vi "menu_song_select.vi"(0 "song id":enum16{"0", "1"}(ring), 1 "difficulty":enum16{"easy", "hard"}(ring), 2 "showcase":bool=TRUE, 3 "state change":bool=TRUE, 4 "game state":T1(ring), 5 "timer":dbl, 6 "prepare menu":enum16{"difficulty", "bot"}(ring)) -> (14 "new picture":picture, 17 "animating?":bool)   [LabVIEW 2023]
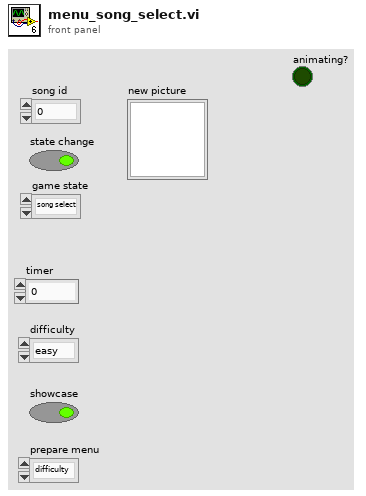
[diagram p1: front panel]
types:
  T1 = enum16{"song select", "difficulty select", "gameplay", "result"}
  T2 = cluster{"Width":i16, "Style":enum32{"Solid", "Dash", "Dot", "DashDot", "DashDotDot"}}
  T3 = cluster{"Width":u16, "Style":enum32{"Solid", "Dash", "Dot", "DashDot", "DashDotDot"}}
  T4 = cluster{"horizontal":enum16{"left", "center", "right"}, "vertical":enum16{"top", "center", "bottom"}}
  T5 = cluster{"Font Name:":string, "Size":i16, "Strikeout?":bool, "Italic?":bool, "Underline?":bool, "Outline?":bool, "Shadow?":bool, "Bold?":bool}
  T6 = enum16{"User-specified Font", "Application Font", "System Font", "Dialog Font"}
  T7 = enum16{"None", "Stacked", "Clockwise", "Counterclockwise"}
  T8 = typedef "imagedata.ctl" = cluster{"image type":i32, "image depth":i32, "image":u8[], "mask":u8[], "colors":u32[], "Rectangle":cluster{"left":i16, "top":i16, "right":i16, "bottom":i16}}
  T9 = cluster{"left":i16, "left":i16, dbl, "bottom":i16}
  T10 = cluster{dbl, "top":i16, "right":i16, "bottom":i16}
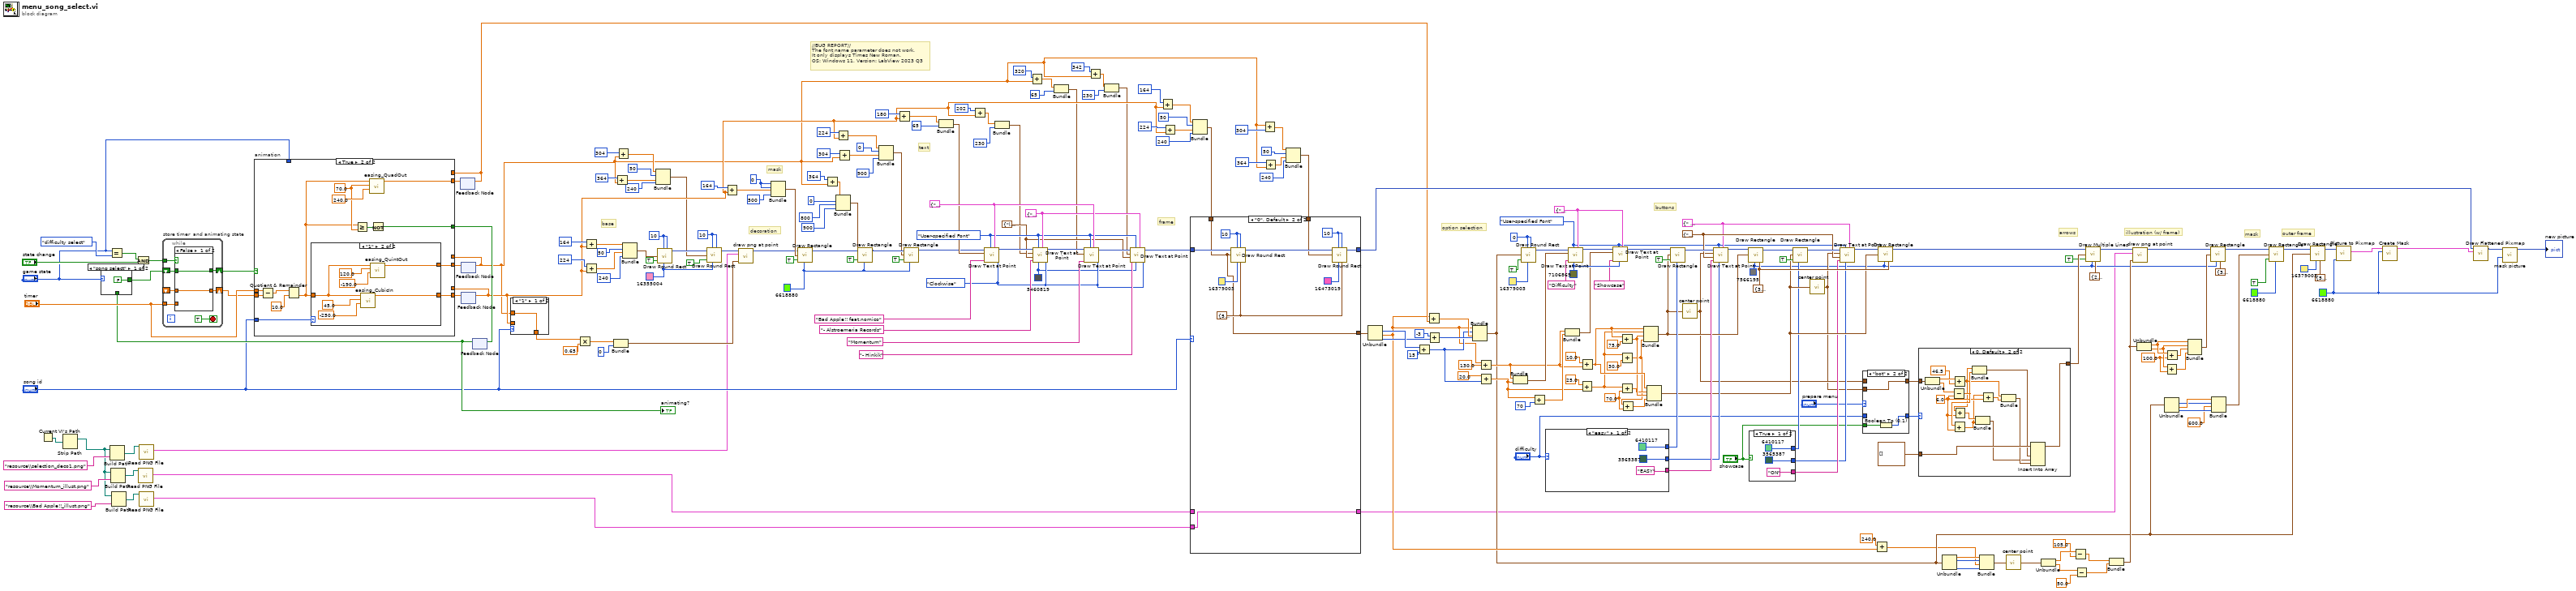
[diagram p0: block diagram]
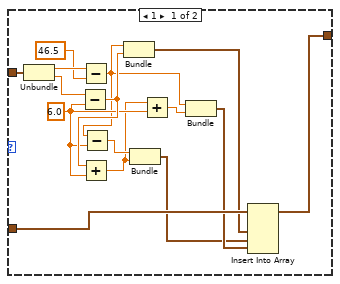
[diagram p2: hidden frame]
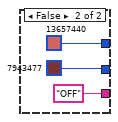
[diagram p4: hidden frame]
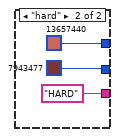
[diagram p5: hidden frame]
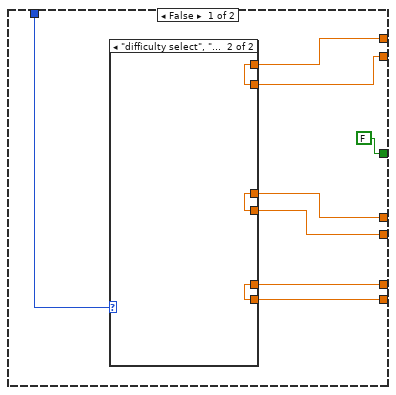
[diagram p7: hidden frame]
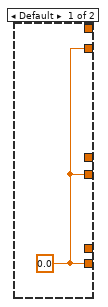
[diagram p8: hidden frame]
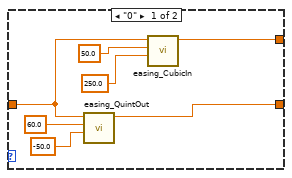
[diagram p9: hidden frame]
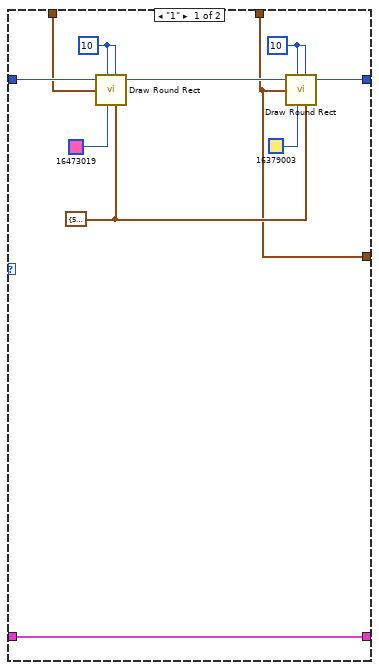
[diagram p12: hidden frame]
diagram:
  w47 = 100.0 ("y")
  w85 = 70.0 ("x")
  w80 = T4 {"horizontal"=enum."center", "vertical"=enum."center"} ("alignment(left, top)")
  w78 = T5 {"Font Name:"=" ", "Size"=15, "Strikeout?"=FALSE, "Italic?"=FALSE, "Underline?"=FALSE, "Outline?"=FALSE, "Shadow?"=FALSE, "Bold?"=TRUE} ("[user-specified font]")
  w81 = T2 {"Width"=3, "Style"=enum."DashDotDot"} ("pen")
  w43 = u32 7566195 ("color(black)")
  w106 = u32 5460819 ("text color(black)")
  w112 = u32 7106869 ("text color(black)")
  w77 = T6."User-specified Font" ("desired font(Application)")
  w113 = T5 {"Font Name:"="a", "Size"=16, "Strikeout?"=FALSE, "Italic?"=FALSE, "Underline?"=FALSE, "Outline?"=FALSE, "Shadow?"=FALSE, "Bold?"=TRUE} ("[user-specified font]")
  w120 = i16 0
  w176 = T7."Clockwise" ("text orientation")
  w197 = i16 0 ("left")
  w221 = T5 {"Font Name:"="k", "Size"=13, "Strikeout?"=FALSE, "Italic?"=TRUE, "Underline?"=FALSE, "Outline?"=FALSE, "Shadow?"=FALSE, "Bold?"=TRUE} ("[user-specified font]")
  w219 = T4 {"horizontal"=enum."left", "vertical"=enum."bottom"} ("alignment(left, top)")
  w222 = T5 {"Font Name:"="Arial", "Size"=15, "Strikeout?"=FALSE, "Italic?"=FALSE, "Underline?"=FALSE, "Outline?"=FALSE, "Shadow?"=FALSE, "Bold?"=TRUE} ("[user-specified font]")
  w220 = T6."User-specified Font" ("desired font(Application)")
  w29 = u32 6618880 ("color(black)")
  w18 = u32 6618880 ("color(black)")
  w235 = i16 10
  w236 = i16 10
  w234 = u32 16355004 ("color(black)")
  # "outer frame"
  # "mask"
  # "illustration (w/ frame)"
  # "arrows"
  # "buttons"
  # "//BUG REPORT//\nThe font name parameter does not work.\nIt only displays Times New Roman.\nOS: Windows 11, Version: LabView 2023 Q3"
  # "option selection"
  # "frame"
  # "text"
  # "mask"
  # "decoration"
  # "base"
  n1 = Current VI's Path() -> (path=w14:path)
  n2 = Strip Path(path=w14) -> (stripped path=w11:path)  [unwired: 1 out]
  n3 = Equal?(x="game state", y=T1."difficulty select" ("game state 2")) -> (x = y?=w215:bool)
  n4 = Build Path(base path=w11, name or relative path="resource\\selection_deco1.png") -> (appended path=w9:path)
  n5 = Build Path(base path=w11, name or relative path="resource\\Momentum_illust.png") -> (appended path=w7:path)
  n6 = Build Path(base path=w11, name or relative path="resource\\Bad Apple!!_illust.png") -> (appended path=w5:path)
  n7 = And(x=w215, y="state change") -> (x .and. y?=w214:bool)
  n8 = call <vilib>:"Read PNG File.vi"("path to PNG file"=w7) -> ("image data"=w6:T8)  [unwired: 8 in, 2 out]
  n9 = call <vilib>:"Read PNG File.vi"("path to PNG file"=w5) -> ("image data"=w4:T8)  [unwired: 8 in, 2 out]
  n10 = call <vilib>:"Read PNG File.vi"("path to PNG file"=w9) -> ("image data"=w8:T8)  [unwired: 8 in, 2 out]
  n11 = feedback #1() -> (w37:dbl)  [unwired: 1 in]
  n12 = feedback #2() -> (w130:dbl)  [unwired: 1 in]
  n13 = feedback #3() -> (w158:dbl)  [unwired: 1 in]
  n14 = feedback #4() -> (w161:bool)  [unwired: 1 in]
  "animating?" <- w161
  n15 = case shown="\"song select\"" "game state" {
    tunnel: [FALSE w240] -> w209
    tunnel: w161 -> [_ w240]
    frame "song select" {
    }
    frame Default {
    }
  }
  n16 = while "store timer  and animating state" {
    tunnel: w214 -> [w246]
    tunnel: "timer" -> [w245]
    shift-right: [w244] -> w210
    shift-left: _ -> [w243]
    shift-right: [w242] -> w203
    shift-left: w209 -> [w241]
    stop <- TRUE stop-if-true
    n17 = case shown="False" w246 {
      selector: w246 -> [_ w250]
      tunnel: w245 -> [_ w251]
      tunnel: [w249 w251] -> w244
      tunnel: w243 -> [w249 _]
      tunnel: [w248 w250] -> w242
      tunnel: w241 -> [w248 _]
      frame False {
      }
      frame True {
      }
    }
  }
  n18 = case "animation" shown="True" w203 {
    tunnel: "timer" -> [_ w276]
    tunnel: w210 -> [_ w275]
    tunnel: [w257 w272] -> w205
    tunnel: w158 -> [w256 _]
    tunnel: [FALSE ("fill?(F)") w264] -> w204
    tunnel: "game state" -> [w258 _]
    tunnel: "song id" -> [_ w271]
    tunnel: [w255 w270] -> w160
    tunnel: w130 -> [w254 _]
    tunnel: [w253 w266] -> w38
    tunnel: w37 -> [w252 _]
    frame False {
      n19 = case shown="\"difficulty select\", \"gameplay\"" w258 {
        tunnel: [w260 w263] -> w257
        tunnel: w256 -> [_ w263]
        tunnel: [w260 w262] -> w255
        tunnel: w254 -> [_ w262]
        tunnel: [w260 w261] -> w253
        tunnel: w252 -> [_ w261]
        frame Default {
          w260 = 0.0
        }
        frame "difficulty select", "gameplay" {
        }
      }
    }
    frame True {
      w268 = 70.0 ("y")
      n20 = Subtract(x=w276, y=w275) -> (x-y=w274:dbl)
      n21 = Quotient & Remainder(x=w274, y=10.0) -> (floor(x/y)=w267:dbl)  [unwired: 1 out]
      n22 = case shown="\"1\"" w271 {
        tunnel: w267 -> [w279 w284]
        tunnel: [w281 w286] -> w272
        tunnel: [w280 w289] -> w270
        frame "0" {
          n23 = call "easing_QuintOut.vi"("distance"=-50.0 ("y"), "interval (10 ms)"=60.0 ("y"), "time"=w279) -> ("current pos"=w281:dbl)  [unwired: 8 in]
          n24 = call "easing_CubicIn.vi"("distance"=250.0 ("y"), "interval (10 ms)"=50.0 ("y"), "time"=w279) -> ("current position"=w280:dbl)  [unwired: 8 in]
        }
        frame "1" {
          n25 = call "easing_CubicIn.vi"("distance"=-250.0 ("y"), "interval (10 ms)"=45.0 ("y"), "time"=w284) -> ("current position"=w286:dbl)  [unwired: 8 in]
          n26 = call "easing_QuintOut.vi"("distance"=-190.0 ("y"), "interval (10 ms)"=120.0 ("y"), "time"=w284) -> ("current pos"=w289:dbl)  [unwired: 8 in]
        }
      }
      n27 = Greater Or Equal?(x=w267, y=w268) -> (x >= y?=w265:bool)
      n28 = call "easing_QuadOut.vi"("distance"=240.0 ("y"), "interval (10 ms)"=w268, "time"=w267) -> ("current pos"=w266:dbl)  [unwired: 8 in]
      n29 = Not(x=w265) -> (.not. x?=w264:bool)
    }
  }
  n30 = feedback-in #1(w38) -> ()
  n31 = feedback-in #2(w160) -> ()
  n32 = feedback-in #3(w205) -> ()
  n33 = feedback-in #4(w204) -> ()
  n34 = case shown="\"1\"" "song id" {
    tunnel: [w291 w292] -> w159
    tunnel: w158 -> [_ w292]
    tunnel: w130 -> [w291 _]
    frame "1" {
    }
    frame "0" {
    }
  }
  n35 = Multiply(x=w159, y=0.65) -> (x*y=w170:dbl)
  n36 = Add(x=i16 164, y=w158) -> (x+y=w198:dbl)
  n37 = Add(x=i16 224, y=w158) -> (x+y=w200:dbl)
  n38 = Bundle(w170, "y"=i16 0) -> (w173:cluster{dbl, "y":i16})  [unwired: 1 in]
  n39 = Add(x=i16 364 ("right"), y=w130) -> (x+y=w151:dbl)
  n40 = Add(x=i16 304 ("left"), y=w130) -> (x+y=w150:dbl)
  n41 = Bundle(w198, i16 50, w200, i16 240) -> (w206:cluster{dbl, i16, dbl, i16})  [unwired: 1 in]
  n42 = Bundle(w150, "top"=i16 50, w151, "bottom"=i16 240) -> (w156:cluster{dbl, "top":i16, dbl, "bottom":i16})  [unwired: 1 in]
  n43 = call <vilib>:"Draw Round Rect.vi"("oval width"=w236, "rect"=w206, "fill?(F)"=TRUE, "color(black)"=w234, "oval height"=w236) -> ("new picture"=w233:picture)  [unwired: 4 in]
  n44 = call <vilib>:"Draw Round Rect.vi"("picture"=w233, "oval width"=w235, "rect"=w156, "fill?(F)"=TRUE, "color(black)"=w234, "oval height"=w235) -> ("new picture"=w174:picture)  [unwired: 3 in]
  n45 = Add(x=i16 164 ("right"), y=w158) -> (x+y=w193:dbl)
  n46 = call "draw png at point.vi"("top left point(0, 0)"=w173, "image data"=w8, "new picture in"=w174) -> ("new picture out"=w175:picture)  [unwired: 8 in]
  n47 = Bundle("left"=w197, "left"=w197, w193, "bottom"=i16 500) -> (w195:T9)  [unwired: 1 in]
  n48 = call <vilib>:"Draw Rectangle.vi"("picture"=w175, "rect"=w195, "fill?(F)"=TRUE, "color(black)"=w29) -> ("new picture"=w230:picture)  [unwired: 5 in]
  n49 = Add(x=i16 364 ("left"), y=w130) -> (x+y=w131:dbl)
  n50 = Add(x=i16 224 ("left"), y=w158) -> (x+y=w177:dbl)
  n51 = Bundle(w131, "top"=i16 0, "right"=i16 800, "bottom"=i16 900) -> (w192:T10)  [unwired: 1 in]
  n52 = Add(x=i16 304 ("right"), y=w130) -> (x+y=w148:dbl)
  n53 = call <vilib>:"Draw Rectangle.vi"("picture"=w230, "rect"=w192, "fill?(F)"=TRUE, "color(black)"=w29) -> ("new picture"=w228:picture)  [unwired: 5 in]
  n54 = Bundle(w177, "top"=i16 0, w148, "bottom"=i16 900) -> (w181:cluster{dbl, "top":i16, dbl, "bottom":i16})  [unwired: 1 in]
  n55 = Add(x=i16 180, y=w158) -> (x+y=w186:dbl)
  n56 = call <vilib>:"Draw Rectangle.vi"("picture"=w228, "rect"=w181, "fill?(F)"=TRUE, "color(black)"=w29) -> ("new picture"=w2:picture)  [unwired: 5 in]
  n57 = Bundle(w186, "y"=i16 65) -> (w188:cluster{dbl, "y":i16})  [unwired: 1 in]
  n58 = Add(x=i16 202, y=w158) -> (x+y=w165:dbl)
  n59 = call <vilib>:"Draw Text at Point.vi"("text orientation"=w176, "[user-specified font]"=w222, "desired font(Application)"=w220, "text"="Bad Apple!! feat.nomico", "origin"=w188, "picture"=w2) -> ("new picture"=w226:picture)  [unwired: 4 in, 1 out]
  n60 = Bundle(w165, "y"=i16 230) -> (w184:cluster{dbl, "y":i16})  [unwired: 1 in]
  n61 = Add(x=i16 320, y=w130) -> (x+y=w144:dbl)
  n62 = call <vilib>:"Draw Text at Point.vi"("text orientation"=w176, "[user-specified font]"=w221, "text color(black)"=w106, "desired font(Application)"=w220, "text"="- Alstroemeria Records", "alignment(left, top)"=w219, "origin"=w184, "picture"=w226) -> ("new picture"=w224:picture)  [unwired: 2 in, 1 out]
  n63 = Bundle(w144, "y"=i16 65) -> (w147:cluster{dbl, "y":i16})  [unwired: 1 in]
  n64 = call <vilib>:"Draw Text at Point.vi"("text orientation"=w176, "[user-specified font]"=w222, "desired font(Application)"=w220, "text"="Momentum", "origin"=w147, "picture"=w224) -> ("new picture"=w223:picture)  [unwired: 4 in, 1 out]
  n65 = Add(x=i16 342, y=w130) -> (x+y=w140:dbl)
  n66 = Bundle(w140, "y"=i16 230) -> (w143:cluster{dbl, "y":i16})  [unwired: 1 in]
  n67 = call <vilib>:"Draw Text at Point.vi"("text orientation"=w176, "[user-specified font]"=w221, "text color(black)"=w106, "desired font(Application)"=w220, "text"="- Hinkik", "alignment(left, top)"=w219, "origin"=w143, "picture"=w223) -> ("new picture"=w216:picture)  [unwired: 2 in, 1 out]
  n68 = Add(x=i16 164 ("left"), y=w158) -> (x+y=w162:dbl)
  n69 = Add(x=i16 224 ("right"), y=w158) -> (x+y=w163:dbl)
  n70 = Bundle(w162, "top"=i16 50, w163, "bottom"=i16 240) -> (w169:cluster{dbl, "top":i16, dbl, "bottom":i16})  [unwired: 1 in]
  n71 = Add(x=w130, y=i16 304 ("left")) -> (x+y=w135:dbl)
  n72 = Add(x=i16 364 ("right"), y=w130) -> (x+y=w133:dbl)
  n73 = Bundle(w135, "top"=i16 50, w133, "bottom"=i16 240) -> (w139:cluster{dbl, "top":i16, dbl, "bottom":i16})  [unwired: 1 in]
  n74 = case shown="\"0\", Default" "song id" {
    tunnel: w216 -> [w303 w314]
    tunnel: [w299 w310] -> w39
    tunnel: w169 -> [w295 w305]
    tunnel: w139 -> [w294 w306]
    tunnel: [w294 w305] -> w127
    tunnel: w6 -> [w293 _]
    tunnel: w4 -> [_ w304]
    tunnel: [w293 w304] -> w3
    frame "1" {
      w296 = i16 10
      w297 = i16 10
      w300 = T3 {"Width"=5, "Style"=enum."Solid"} ("pen")
      n75 = call <vilib>:"Draw Round Rect.vi"("picture"=w303, "oval width"=w297, "rect"=w295, "color(black)"=u32 16473019, "oval height"=w297, "pen"=w300) -> ("new picture"=w302:picture)  [unwired: 3 in]
      n76 = call <vilib>:"Draw Round Rect.vi"("picture"=w302, "oval width"=w296, "rect"=w294, "color(black)"=u32 16379003, "oval height"=w296, "pen"=w300) -> ("new picture"=w299:picture)  [unwired: 3 in]
    }
    frame "0", Default {
      w307 = i16 10
      w308 = i16 10
      w311 = T3 {"Width"=5, "Style"=enum."Solid"} ("pen")
      n77 = call <vilib>:"Draw Round Rect.vi"("picture"=w314, "oval width"=w308, "rect"=w305, "color(black)"=u32 16379003, "oval height"=w308, "pen"=w311) -> ("new picture"=w313:picture)  [unwired: 3 in]
      n78 = call <vilib>:"Draw Round Rect.vi"("picture"=w313, "oval width"=w307, "rect"=w306, "color(black)"=u32 16473019, "oval height"=w307, "pen"=w311) -> ("new picture"=w310:picture)  [unwired: 3 in]
    }
  }
  n79 = Unbundle(w127) -> ("top"=w126:i16, w33:dbl, "bottom"=w123:i16)  [unwired: 1 out]
  n80 = Add(x=w126, y=15) -> (x+y=w110:i32)
  n81 = Add(x=w33, y=w37) -> (x+y=w124:dbl)
  n82 = Add(x=-3, y=w123) -> (x+y=w121:i32)
  n83 = Bundle(w33, w110, w124, w121) -> (w26:cluster{dbl, i32, dbl, i32})  [unwired: 1 in]
  n84 = Add(x=w33, y=130.0) -> (x+y=w100:dbl)
  n85 = Add(x=20.0, y=w110) -> (x+y=w76:dbl)
  n86 = Bundle(w100, w76) -> (w118:cluster{dbl, dbl})  [unwired: 1 in]
  n87 = call <vilib>:"Draw Round Rect.vi"("oval width"=w120, "rect"=w26, "fill?(F)"=TRUE, "color(black)"=u32 16379003, "oval height"=w120) -> ("new picture"=w119:picture)  [unwired: 4 in]
  n88 = Add(x=w76, y=70) -> (x+y=w108:dbl)
  n89 = case shown="\"easy\"" "difficulty" {
    tunnel: [u32 6410117 ("color(black)") u32 13657440 ("color(black)")] -> w96
    tunnel: ["EASY" ("text") "HARD" ("text")] -> w95
    tunnel: [u32 3565387 ("color(black)") u32 7943477 ("color(black)")] -> w93
    frame "easy" {
    }
    frame "hard" {
    }
  }
  n90 = Bundle(w100, w108) -> (w107:cluster{dbl, dbl})  [unwired: 1 in]
  n91 = call <vilib>:"Draw Text at Point.vi"("[user-specified font]"=w113, "text color(black)"=w112, "desired font(Application)"=w77, "text"="Difficulty", "origin"=w118, "picture"=w119) -> ("new picture"=w114:picture)  [unwired: 4 in, 1 out]
  n92 = Add(x=25.0, y=w76) -> (x+y=w88:dbl)
  n93 = Add(x=10.0, y=w100) -> (x+y=w90:dbl)
  n94 = call <vilib>:"Draw Text at Point.vi"("[user-specified font]"=w113, "text color(black)"=w112, "desired font(Application)"=w77, "text"="Showcase", "origin"=w107, "picture"=w114) -> ("new picture"=w105:picture)  [unwired: 4 in, 1 out]
  n95 = Add(x=w90, y=75.0 ("x")) -> (x+y=w89:dbl)
  n96 = Add(x=w88, y=30.0 ("x")) -> (x+y=w86:dbl)
  n97 = Add(x=w88, y=w85) -> (x+y=w87:dbl)
  n98 = Add(x=w86, y=w85) -> (x+y=w84:dbl)
  n99 = Bundle(w90, w88, w89, w86) -> (w94:cluster{dbl, dbl, dbl, dbl})  [unwired: 1 in]
  n100 = Bundle(w90, w87, w89, w84) -> (w79:cluster{dbl, dbl, dbl, dbl})  [unwired: 1 in]
  n101 = call <vilib>:"Draw Rectangle.vi"("picture"=w105, "rect"=w94, "fill?(F)"=TRUE, "color(black)"=w96) -> ("new picture"=w98:picture)  [unwired: 5 in]
  n102 = call "center point.vi"("border"=w94) -> ("center"=w71:cluster{dbl, dbl})  [unwired: 4 in]
  n103 = call <vilib>:"Draw Text at Point.vi"("[user-specified font]"=w78, "text color(black)"=w93, "desired font(Application)"=w77, "text"=w95, "alignment(left, top)"=w80, "origin"=w71, "picture"=w98) -> ("new picture"=w97:picture)  [unwired: 3 in, 1 out]
  n104 = call <vilib>:"Draw Rectangle.vi"("picture"=w97, "rect"=w94, "color(black)"=w43, "pen"=w81) -> ("new picture"=w92:picture)  [unwired: 5 in]
  n105 = case shown="True" "showcase" {
    tunnel: [u32 6410117 ("color(black)") u32 13657440 ("color(black)")] -> w75
    tunnel: ["ON" ("text") "OFF" ("text")] -> w74
    tunnel: [u32 3565387 ("color(black)") u32 7943477 ("color(black)")] -> w73
    frame True {
    }
    frame False {
    }
  }
  n106 = call <vilib>:"Draw Rectangle.vi"("picture"=w92, "rect"=w79, "fill?(F)"=TRUE, "color(black)"=w75) -> ("new picture"=w83:picture)  [unwired: 5 in]
  n107 = call "center point.vi"("border"=w79) -> ("center"=w70:cluster{dbl, dbl})  [unwired: 4 in]
  n108 = call <vilib>:"Draw Text at Point.vi"("[user-specified font]"=w78, "text color(black)"=w73, "desired font(Application)"=w77, "text"=w74, "alignment(left, top)"=w80, "origin"=w70, "picture"=w83) -> ("new picture"=w82:picture)  [unwired: 3 in, 1 out]
  n109 = case shown="\"bot\"" "prepare menu" {
    tunnel: w71 -> [w328 _]
    tunnel: w70 -> [_ w331]
    tunnel: [w328 w331] -> w66
    tunnel: "showcase" -> [_ w330]
    tunnel: [w327 w329] -> w67
    tunnel: "difficulty" -> [w327 _]
    frame "difficulty" {
    }
    frame "bot" {
      n110 = Boolean To (0,1)(Boolean=w330) -> (0, 1=w329:i16)
    }
  }
  n111 = Add(x=240.0 ("y"), y=w33) -> (x+y=w15:dbl)
  n112 = call <vilib>:"Draw Rectangle.vi"("picture"=w82, "rect"=w79, "color(black)"=w43, "pen"=w81) -> ("new picture"=w63:picture)  [unwired: 5 in]
  n113 = case shown="0, Default" w67 {
    tunnel: w66 -> [w346 w361]
    tunnel: cluster{"x":i16, "y":i16}[] [] ("line endpoints") -> [w340 w355]
    tunnel: [w335 w350] -> w64
    frame 1 {
      w339 = 6.0 ("y")
      n114 = Unbundle(w346) -> (w345:dbl, w343:dbl)
      n115 = Subtract(x=w343, y=w339) -> (x-y=w342:dbl)
      n116 = Subtract(x=w345, y=46.5) -> (x-y=w336:dbl)
      n117 = Add(x=w342, y=w339) -> (x+y=w338:dbl)
      n118 = Subtract(x=w336, y=w339) -> (x-y=w341:dbl)
      n119 = Bundle(w336, w342) -> (w332:cluster{dbl, dbl})  [unwired: 1 in]
      n120 = Bundle(w341, w338) -> (w333:cluster{dbl, dbl})  [unwired: 1 in]
      n121 = Add(x=w338, y=w339) -> (x+y=w337:dbl)
      n122 = Bundle(w336, w337) -> (w334:cluster{dbl, dbl})  [unwired: 1 in]
      n123 = Insert Into Array(array=w340, new element #1=w332, new element #2=w333, new element #3=w334) -> (w335:cluster{"x":i16, "y":i16}[])  [unwired: 1 in]
    }
    frame 0, Default {
      w354 = 6.0 ("y")
      n124 = Unbundle(w361) -> (w360:dbl, w358:dbl)
      n125 = Subtract(x=w358, y=w354) -> (x-y=w357:dbl)
      n126 = Add(x=w360, y=46.5) -> (x+y=w351:dbl)
      n127 = Add(x=w357, y=w354) -> (x+y=w353:dbl)
      n128 = Add(x=w351, y=w354) -> (x+y=w356:dbl)
      n129 = Bundle(w351, w357) -> (w347:cluster{dbl, dbl})  [unwired: 1 in]
      n130 = Bundle(w356, w353) -> (w348:cluster{dbl, dbl})  [unwired: 1 in]
      n131 = Add(x=w353, y=w354) -> (x+y=w352:dbl)
      n132 = Bundle(w351, w352) -> (w349:cluster{dbl, dbl})  [unwired: 1 in]
      n133 = Insert Into Array(array=w355, new element #1=w347, new element #2=w348, new element #3=w349) -> (w350:cluster{"x":i16, "y":i16}[])  [unwired: 1 in]
    }
  }
  n134 = Unbundle(w26) -> (w16:dbl, w36:i32, w35:i32)  [unwired: 1 out]
  n135 = Bundle(w16, w36, w15, w35) -> (w34:cluster{dbl, i32, dbl, i32})  [unwired: 1 in]
  n136 = call "center point.vi"("border"=w34) -> ("center"=w60:cluster{dbl, dbl})  [unwired: 4 in]
  n137 = Unbundle(w60) -> (w59:dbl, w56:dbl)
  n138 = Subtract(x=w59, y=105.0) -> (x-y=w57:dbl)
  n139 = Subtract(x=w56, y=50.0) -> (x-y=w54:dbl)
  n140 = call <vilib>:"Draw Multiple Lines.vi"("picture"=w63, "line endpoints"=w64, "fill?(F)"=TRUE, "color(black)"=w43, "pen"=T3 {"Width"=2, "Style"=enum."Solid"}) -> ("new picture"=w53:picture)  [unwired: 4 in]
  n141 = Bundle(w57, w54) -> (w51:cluster{dbl, dbl})  [unwired: 1 in]
  n142 = call "draw png at point.vi"("top left point(0, 0)"=w51, "image data"=w3, "new picture in"=w53) -> ("new picture out"=w52:picture)  [unwired: 8 in]
  n143 = Unbundle(w51) -> (w50:dbl, w48:dbl)
  n144 = Add(x=w48, y=w47) -> (x+y=w46:dbl)
  n145 = Unbundle(w26) -> (w24:i32, w25:dbl, w23:i32)  [unwired: 1 out]
  n146 = Add(x=w50, y=w47) -> (x+y=w49:dbl)
  n147 = Bundle(w50, w48, w49, w46) -> (w45:cluster{dbl, dbl, dbl, dbl})  [unwired: 1 in]
  n148 = call <vilib>:"Draw Rectangle.vi"("picture"=w52, "rect"=w45, "color(black)"=w43, "pen"=T2 {"Width"=3, "Style"=enum."Solid"}) -> ("new picture"=w30:picture)  [unwired: 5 in]
  n149 = Bundle(w25, w24, "y"=600.0, w23) -> (w21:cluster{dbl, i32, "y":dbl, i32})  [unwired: 1 in]
  n150 = call <vilib>:"Draw Rectangle.vi"("picture"=w30, "rect"=w21, "fill?(F)"=TRUE, "color(black)"=u32 6618880) -> ("new picture"=w20:picture)  [unwired: 5 in]
  n151 = call <vilib>:"Draw Rectangle.vi"("picture"=w20, "rect"=w26, "color(black)"=u32 16379003, "pen"=T2 {"Width"=5, "Style"=enum."Solid"}) -> ("new picture"=w31:picture)  [unwired: 5 in]
  n152 = call <vilib>:"Picture to Pixmap.vi"("Background Color"=w18, "picture"=w31) -> ("image data"=w19:T8)  [unwired: 8 in, 1 out]
  n153 = call <vilib>:"Create Mask.vi"("Mask Color (Black)"=w18, "image data"=w19) -> ("image data"=w17:T8)  [unwired: 9 in]
  n154 = call <vilib>:"Draw Flattened Pixmap.vi"("image data"=w17, "picture"=w39) -> ("new picture"=w40:picture)  [unwired: 7 in]
  n155 = call "mask picture.vi"("mask color"=w18, "new picture in"=w40) -> ("new picture out"=→"new picture":picture)  [unwired: 9 in]
